vi "ESP8266_DS18B20_Wifi_LabVIEW2.vi"() -> ()   [LabVIEW 2018]
uses:
  4235e3a1-d292-4cba-9d32-bc6c7079b231.vi
  b0b94500-097e-4b2b-a1a6-b2d27f4505f2.vi
  <vilib>/httpClient/LabVIEWHTTPClient.lvlib
panel:
  out "current temp2":string
  out "temp2 array":dbl[](array[numeric])
  out "Temp2 Graph":dbl[](graph)
  out "value cluster":T1
  in  "milliseconds to wait":u32=30000
  out "Temp1 Graph":dbl[](graph)
  out "temp1 array":dbl[](array[numeric])
  out "current temp1":string
  in  "Format ref cluster":T1
  in  "stop":bool
  out "body":string
  out "headers":string
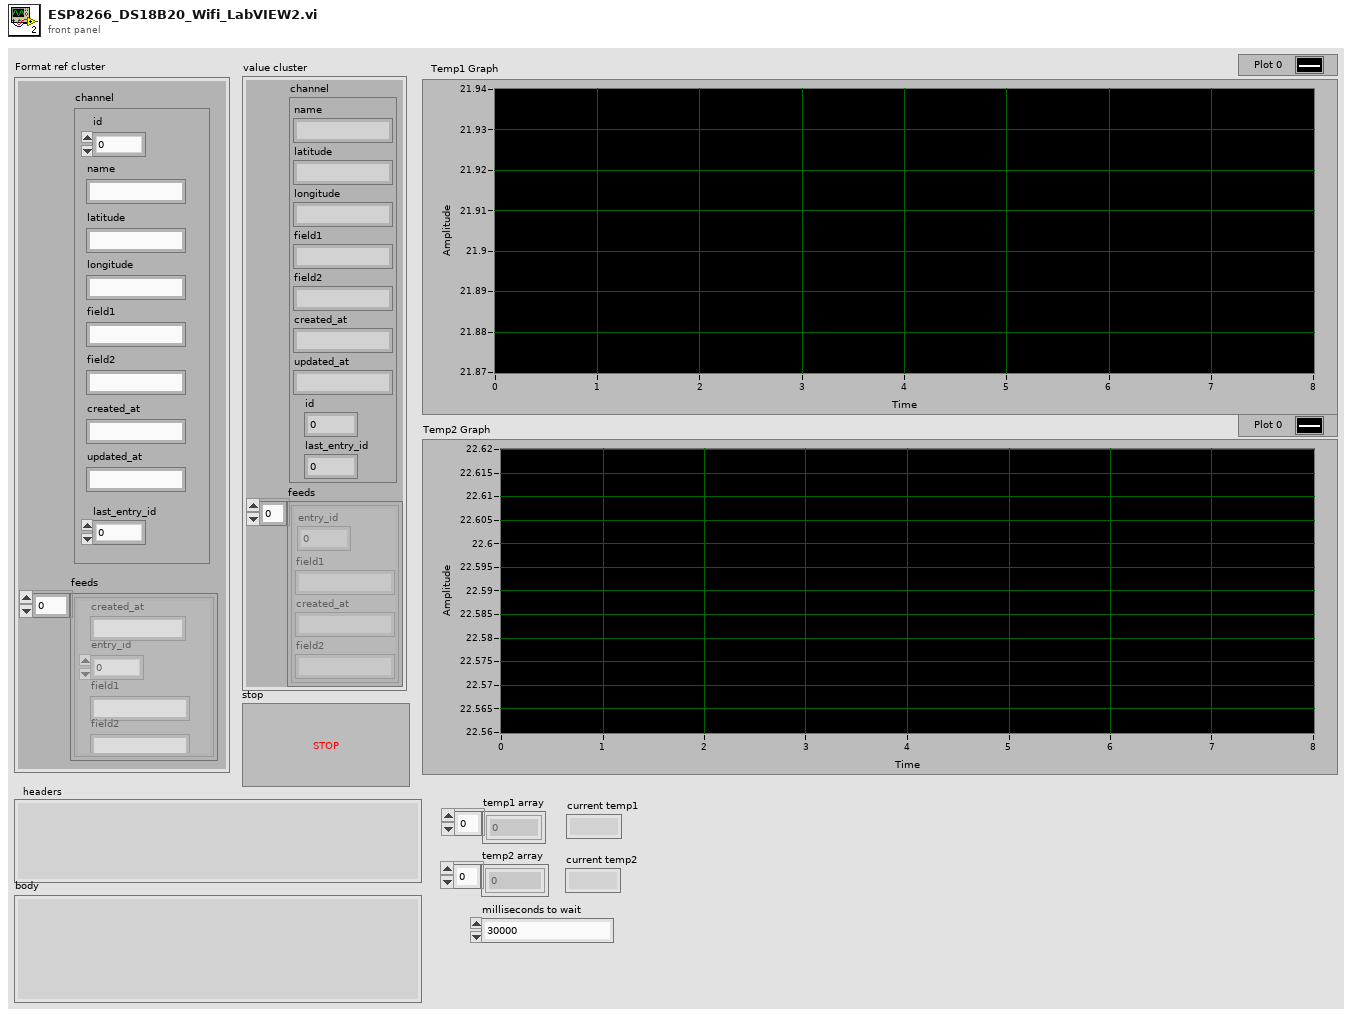
[diagram p1: front panel]
types:
  T1 = cluster{"channel":cluster{"name":string, "latitude":string, "longitude":string, "field1":string, "field2":string, "created_at":string, "updated_at":string, "id":dbl, "last_entry_id":dbl}, "feeds":cluster{"entry_id":dbl, "field1":string, "created_at":string, "field2":string}[]}
  T2 = typedef "LabVIEWHTTPClient.lvlib/ClientHandle.ctl" = refnum<k1>
  T3 = cluster{"entry_id":dbl, "field1":string, "created_at":string, "field2":string}[]
  T4 = cluster{"entry_id":dbl, "field1":string, "created_at":string, "field2":string}
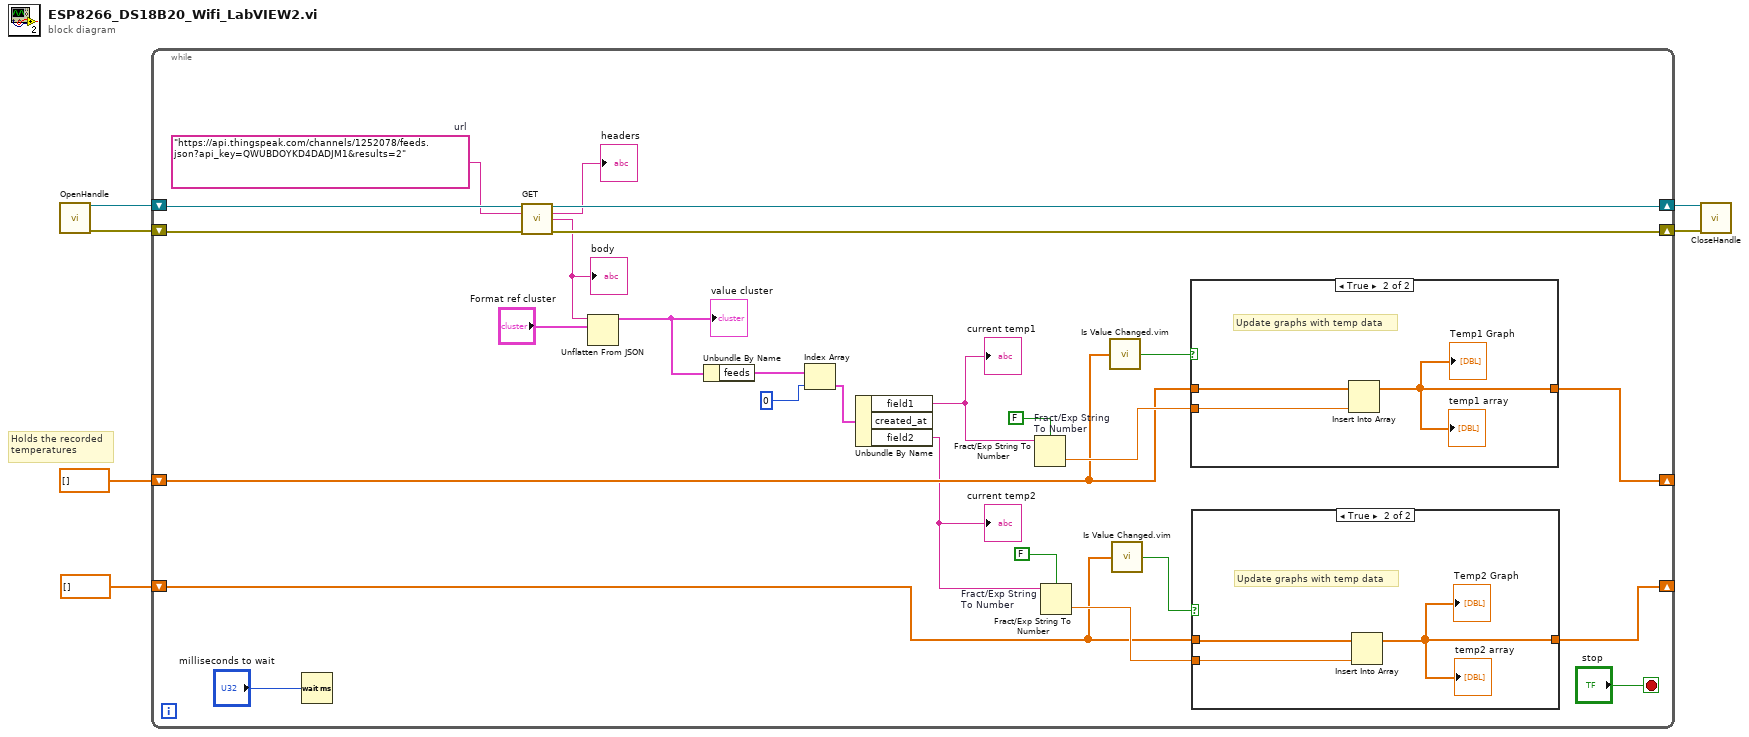
[diagram p0: block diagram]
diagram:
  # "Holds the recorded\ntemperatures"
  n1 = call <vilib>:"OpenHandle.vi"() -> ("client handle out"=w6:T2, "error out"=w4:errorcluster)  [unwired: 14 in]
  n2 = while {
    shift-right: [w30] -> w5
    shift-left: w6 -> [w32]
    shift-right: [w28] -> w3
    shift-left: w4 -> [w29]
    shift-right: [w15] -> _
    shift-left: dbl[] [] -> [w13]
    shift-right: [w9] -> _
    shift-left: dbl[] [] -> [w7]
    stop <- "stop" stop-if-true
    w31 = "https://api.thingspeak.com/channels/1252078/feeds.json?api_key=QWUBDOYKD4DADJM1&results=2"  # url
    n3 = Wait (ms)(milliseconds to wait="milliseconds to wait") -> ()  [unwired: 1 out]
    n4 = call <vilib>:"GET.vi"("client handle"=w32, "url"=w31, "error in (no error)"=w29) -> ("client handle out"=w30:T2, "headers"=→"headers":string, "body"=w24:string, "error out"=w28:errorcluster)  [unwired: 9 in]
    "body" <- w24
    n5 = Unflatten From JSON(JSON string=w24, type and defaults="Format ref cluster") -> (value=w22:T1)  [unwired: 5 in, 1 out]
    "value cluster" <- w22
    n6 = Unbundle By Name "Unbundle By Name"(w22) -> ("feeds"=w20:T3)
    n7 = Index Array "Index Array"(array=w20, index=0) -> (element=w19:T4)
    n8 = Unbundle By Name "Unbundle By Name"(w19) -> ("field1"=w18:string, "field2"=w11:string)  [unwired: 1 out]
    "current temp1" <- w18
    "current temp2" <- w11
    n9 = Fract/Exp String To Number "Fract/Exp String \nTo Number"(use system decimal point (T)=FALSE, string=w18) -> (number=w16:dbl)  [unwired: 2 in, 1 out]
    n10 = Fract/Exp String To Number "Fract/Exp String \nTo Number"(use system decimal point (T)=FALSE, string=w11) -> (number=w10:dbl)  [unwired: 2 in, 1 out]
    n11 = call "Is Value Changed.vim"("value"=w13) -> ("changed or first call?"=w14:bool)
    n12 = call "Is Value Changed.vim"("value"=w7) -> ("changed or first call?"=w8:bool)
    n13 = case shown="True" w14 {
      tunnel: w16 -> [_ w40]
      tunnel: w13 -> [w37 w39]
      tunnel: [w37 w38] -> w15
      frame False {
      }
      frame True {
        # "Update graphs with temp data"
        n14 = Insert Into Array "Insert Into Array"(array=w39, new element=w40) -> (w38:dbl[])  [unwired: 1 in]
        "Temp1 Graph" <- w38
        "temp1 array" <- w38
      }
    }
    n15 = case shown="True" w8 {
      tunnel: w7 -> [w33 w36]
      tunnel: w10 -> [_ w35]
      tunnel: [w33 w34] -> w9
      frame False {
      }
      frame True {
        # "Update graphs with temp data"
        n16 = Insert Into Array "Insert Into Array"(array=w36, new element=w35) -> (w34:dbl[])  [unwired: 1 in]
        "Temp2 Graph" <- w34
        "temp2 array" <- w34
      }
    }
  }
  n17 = call <vilib>:"CloseHandle.vi"("client handle"=w5, "error in (no error)"=w3) -> ()  [unwired: 13 in, 1 out]
